vi "Throw Event.vi"(8 "error in (no error)":errorcluster, 10 "Panel Event":T1, 11 "Controller in":refnum<class "Panel Helper.lvclass">) -> (0 "error out":errorcluster)   [LabVIEW 2019, in "Panel.lvlib" / "Panel Helper.lvclass"]
doc: "Throws a panel event.\n----\nCopyright: MGI 2017\nAuthor: Derek Trepanier"
uses:
  <vilib>/MGI/Panel Manager/Panel/Panel Helper/Panel Helper.lvclass
  <vilib>/MGI/Panel Manager/Panel/Panel Helper/Events.ctl
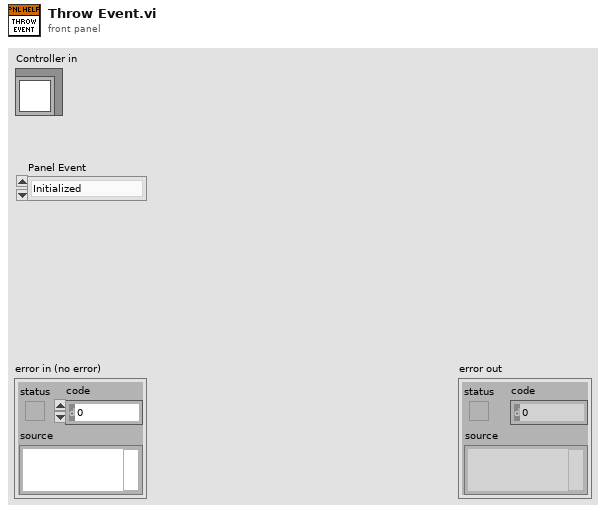
[diagram p1: front panel]
types:
  T1 = typedef "Panel.lvlib/Panel Helper.lvclass/Events.ctl" = enum16{"Initialized", "Shown", "Hidden", "Closed"}
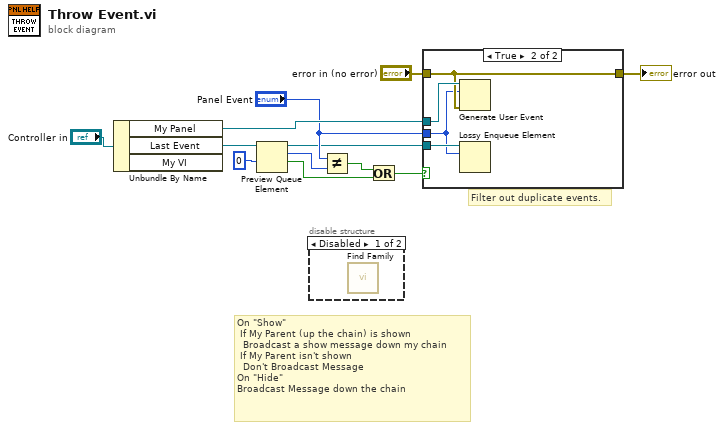
[diagram p0: block diagram]
diagram:
  # "On \"Show\"\n\tIf My Parent (up the chain) is shown\n\t\tBroadcast a show message down my chain\n\tIf My Parent isn't shown\n\t\tDon't Broadcast Message\nOn \"Hide\"\nBroadcast Message down the chain"
  # "Filter out duplicate events."
  n1 = Unbundle By Name("Controller in") -> ("My Panel"=w11:refnum<user-event>, "Last Event"=w9:refnum<queue>)  [unwired: 1 out]
  n2 = Preview Queue Element(queue=w9, timeout in ms (-1)=0) -> (queue out=w1:refnum<queue>, element=w7:T1, timed out?=w4:bool)  [unwired: 1 in, 1 out]
  n3 = disable-structure shown="Disabled" {
    frame Disabled {
      n4 = call "Find Family.vi"() -> ()  [unwired: 9 in, 3 out]
    }
    frame Enabled {
    }
  }
  n5 = Not Equal?(x="Panel Event", y=w7) -> (x != y?=w5:bool)
  n6 = Or(x=w5, y=w4) -> (x .or. y?=w3:bool)
  n7 = case shown="True" w3 {
    tunnel: w11 -> [_ w17]
    tunnel: "error in (no error)" -> [w13 w16]
    tunnel: "Panel Event" -> [_ w14]
    tunnel: [w13 w16] -> w2
    tunnel: w1 -> [_ w15]
    frame False {
    }
    frame True {
      n8 = Generate User Event(user event=w17, event data cluster=w14, error in=w16) -> ()  [unwired: 1 in, 2 out]
      n9 = Lossy Enqueue Element(queue=w15, element=w14) -> ()  [unwired: 1 in, 4 out]
    }
  }
  "error out" <- w2
